vi "MT Generate Symbol Map.vi"   [LabVIEW 2020, in "niDMT.lvlib"]
doc: "Generates an arbitrarily shaped symbol map representing the I/Q constellation points. Use this VI to generate either rectangular or circular I/Q symbol maps."
uses:
  <vilib>/addons/Modulation/niDMT.lvlib
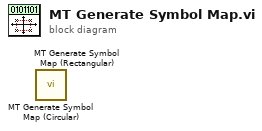
[diagram p0: block diagram]
diagram:
  n1 = call <vilib>:"MT Generate Symbol Map (Circular).vi"() -> ()  [unwired: 14 in, 2 out]
  n2 = call <vilib>:"MT Generate Symbol Map (Rectangular).vi"() -> ()  [unwired: 14 in, 2 out]
